vi "setScript.vi"(8 "error in (no error)":errorcluster, 10 "Script":string, 11 "tBSONJavaScript in":refnum<class "tBSONJavaScript.lvclass">) -> (0 "error out":errorcluster, 3 "tBSONJavaScript out":refnum<class "tBSONJavaScript.lvclass">)   [LabVIEW 2013, in "BSON.lvlib" / "tBSONJavaScript.lvclass"]
uses:
  tBSONJavaScript.lvclass
  tBSONJavaScript.lvclass/tBSONJavaScript.ctl
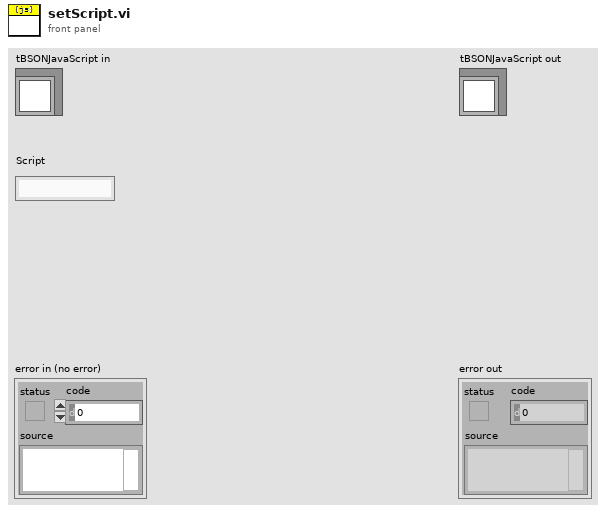
[diagram p1: front panel]
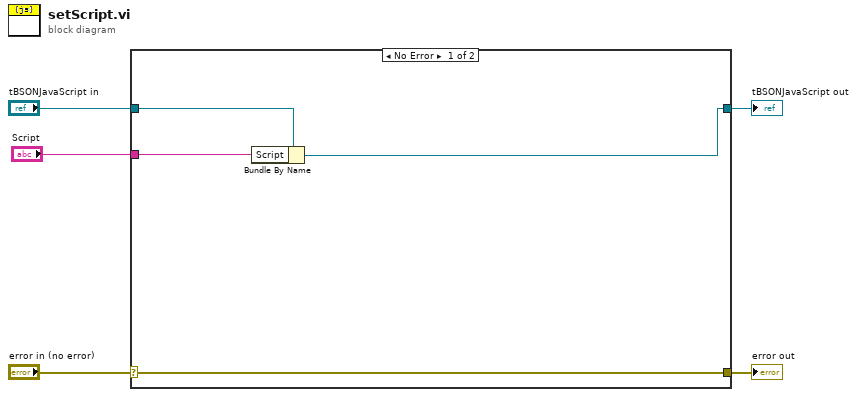
[diagram p0: block diagram]
diagram:
  n1 = case shown="No Error" "error in (no error)" {
    selector: "error in (no error)" -> [w9 w11]
    tunnel: [w9 w11] -> w4
    tunnel: [w6 w10] -> w2
    tunnel: "tBSONJavaScript in" -> [w8 w10]
    tunnel: "Script" -> [w7 _]
    frame No Error {
      n2 = Bundle By Name(cluster=w8, "Script"=w7) -> (w6:refnum<class "tBSONJavaScript.lvclass">)
    }
    frame Error {
    }
  }
  "error out" <- w4
  "tBSONJavaScript out" <- w2
